vi "MGCC_LoadFcst_main.vi"() -> ()   [LabVIEW 2016]
uses:
  Sub-VIs/LoadCombinations.vi
  Sub-VIs/SW_Combinations.vi
  Sub-VIs/CriticalLoadIndex.vi
  <vilib>/imath/engines/lvmath2/RunTimeEngine/IndexRead/NIMS M($,S).vi
  <instcachedir>/0/NIMS M($,S)_3E5749BBB62E49528D4765A77F1F6D98.lvgen/NIMS M($,S)_3E5749BBB62E49528D4765A77F1F6D98_000.vi
  <vilib>/imath/engines/lvmath2/RunTimeEngine/BuiltInFunctions/findnz/NIMS_[1o]_findnz(GColV).vi
  <instcachedir>/0/NIMS_[1o]_findnz(GColV)_8556557C9365446B906472366DD9B2D8.lvgen/NIMS_[1o]_findnz(GColV)_8556557C9365446B906472366DD9B2D8_000.vi
  <vilib>/imath/engines/lvmath2/RunTimeEngine/BuiltInFunctions/length/NIMS_length(GV).vi
  <instcachedir>/0/NIMS_length(GV)_08A3D13377FD4E4B96F5795FBF3698FA.lvgen/NIMS_length(GV)_08A3D13377FD4E4B96F5795FBF3698FA_002.vi
  <vilib>/imath/engines/lvmath2/RunTimeEngine/ErrorHandling/NIMS_Create Error From Enums.vi
  <instcachedir>/0/NIMS_length(GV)_08A3D13377FD4E4B96F5795FBF3698FA.lvgen/NIMS_length(GV)_08A3D13377FD4E4B96F5795FBF3698FA_000.vi
  <vilib>/imath/engines/lvmath2/RunTimeEngine/BuiltInFunctions/zeros/NIMS_M=zeros(I32,I32).vi
  <vilib>/imathl/engines/lvmath/Functions/Error Handling/Create Error.vi
  <vilib>/imath/engines/lvmath2/RunTimeEngine/RangeToken/NIMS_Range_R2 - Integer.vi
  <instcachedir>/0/NIMS_Range_R2 - Integer_89B873E74E6E489885E44F751DD9C6BF.lvgen/NIMS_Range_R2 - Integer_89B873E74E6E489885E44F751DD9C6BF_000.vi
  <vilib>/imath/engines/lvmath2/RunTimeEngine/CommandStatement/MC_CommandStatement_break.vi
  <vilib>/imath/engines/lvmath2/RunTimeEngine/IndexRead/NIMS V(S).vi
  <instcachedir>/0/NIMS V(S)_0488751826AF41519A22953C041130DC.lvgen/NIMS V(S)_0488751826AF41519A22953C041130DC_000.vi
  <vilib>/imath/engines/lvmath2/RunTimeEngine/BuiltInFunctions/is_empty/NIMS_is_empty(GV).vi
  <instcachedir>/0/NIMS_is_empty(GV)_FC7E7C3D9544432CB6AA2416ADCF6D56.lvgen/NIMS_is_empty(GV)_FC7E7C3D9544432CB6AA2416ADCF6D56_000.vi
  <instcachedir>/0/NIMS V(S)_0488751826AF41519A22953C041130DC.lvgen/NIMS V(S)_0488751826AF41519A22953C041130DC_002.vi
  <vilib>/imath/engines/lvmath2/RunTimeEngine/IndexReplace/NIMS M(S,S)=S.vi
  <instcachedir>/0/NIMS M(S,S)=S_98E40400474E4398B113AE20298B4F82.lvgen/NIMS M(S,S)=S_98E40400474E4398B113AE20298B4F82_002.vi
  <vilib>/imath/engines/lvmath2/RunTimeEngine/NodeEndStatement/NIMS_NodeEndStatement_Output.vi
  <instcachedir>/0/NIMS_NodeEndStatement_Output_53EC0D466D134D7ABD903AC30B43404B.lvgen/NIMS_NodeEndStatement_Output_53EC0D466D134D7ABD903AC30B43404B_010.vi
  <vilib>/imath/engines/lvmath2/RunTimeEngine/ErrorHandling/NIMS_Finalize Error.vi
  Finite State Machine/Sub-VIs/MGCC_FntStaMach_gobal.vi
  <vilib>/Utility/error.llb/Error Cluster From Error Code.vi
  Communication/Global communication.vi
  Sub-VIs/Load_Mode.vi
  <vilib>/imath/engines/lvmath2/RunTimeEngine/Managers/WorkSpace/UID Generator.vi
  <vilib>/imath/engines/lvmath2/RunTimeEngine/ArithmeticOperatorToken/NIMS_ArithmeticOperator_times.vi
  <instcachedir>/0/NIMS_ArithmeticOperator_times_953B34F74CAC448FB707D816A29CC5F0.lvgen/NIMS_ArithmeticOperator_times_953B34F74CAC448FB707D816A29CC5F0_000.vi
  <vilib>/imath/engines/lvmath2/RunTimeEngine/ArithmeticOperatorToken/NIMS_ArithmeticOperator_multmx(M,CV).vi
  <instcachedir>/0/NIMS_ArithmeticOperator_multmx(M,CV)_EE734FC8520844C9A7CC1A67008668A3.lvgen/NIMS_ArithmeticOperator_multmx(M,CV)_EE734FC8520844C9A7CC1A67008668A3_001.vi
  <vilib>/imath/engines/lvmath2/RunTimeEngine/BuiltInFunctions/length/NIMS_length(GM).vi
  <instcachedir>/0/NIMS_length(GM)_47CEC356FCE0482D9BA47DC61C99F2C7.lvgen/NIMS_length(GM)_47CEC356FCE0482D9BA47DC61C99F2C7_000.vi
  <vilib>/imath/engines/lvmath2/RunTimeEngine/IndexRead/NIMS M(S).vi
  <instcachedir>/0/NIMS M(S)_B826C018497E4940AE96BD27B540B6FB.lvgen/NIMS M(S)_B826C018497E4940AE96BD27B540B6FB_000.vi
  <vilib>/imath/engines/lvmath2/RunTimeEngine/BuiltInFunctions/is_empty/NIMS_is_empty(GM).vi
  <instcachedir>/0/NIMS_is_empty(GM)_AF8F13F4B7FD436CB1855477E2504B8A.lvgen/NIMS_is_empty(GM)_AF8F13F4B7FD436CB1855477E2504B8A_004.vi
  <vilib>/imath/engines/lvmath2/RunTimeEngine/IndexReplace/NIMS M(S)=S.vi
  <instcachedir>/0/NIMS M(S)=S_B3274CDAFA9346529812A4A947D623CC.lvgen/NIMS M(S)=S_B3274CDAFA9346529812A4A947D623CC_001.vi
  <vilib>/imath/engines/lvmath2/RunTimeEngine/RunTimeType/NIMS_RunTimeType_From StrictType (excl LVString).vi
  <instcachedir>/0/NIMS_RunTimeType_From StrictType (excl LVString)_BBF44FB49F834B71AF7A14CCEDF8BECD.lvgen/NIMS_RunTimeType_From StrictType (excl LVString)_BBF44FB49F834B71AF7A14CCEDF8BECD_000.vi
  <vilib>/imath/engines/lvmath2/RunTimeEngine/LocalVariableDefStatement/MC_LocalVariableDefStatement_Display.vi
  <vilib>/imath/engines/lvmath2/RunTimeEngine/BuiltInFunctions/size/NIMS_[I32,I32]=size(GM).vi
  <instcachedir>/0/NIMS_[I32,I32]=size(GM)_B0A6EC1255BB4C8AB801FE6F734128D9.lvgen/NIMS_[I32,I32]=size(GM)_B0A6EC1255BB4C8AB801FE6F734128D9_000.vi
  <vilib>/imath/engines/lvmath2/RunTimeEngine/IndexRead/NIMS M(S,S).vi
  <instcachedir>/0/NIMS M(S,S)_AC51E74150A542F7991B9634C66F3096.lvgen/NIMS M(S,S)_AC51E74150A542F7991B9634C66F3096_000.vi
  <vilib>/imath/engines/lvmath2/RunTimeEngine/Managers/SymbolTable/Clear UID.vi
  <instcachedir>/0/NIMS_NodeEndStatement_Output_53EC0D466D134D7ABD903AC30B43404B.lvgen/NIMS_NodeEndStatement_Output_53EC0D466D134D7ABD903AC30B43404B_002.vi
  <vilib>/ErrorRing/Error Ring.xnode
  <vilib>/Analysis/NI_AALBase.lvlib
  <vilib>/imath/engines/lvmath2/RunTimeEngine/Managers/SymbolTable/NIMS_WorkSpace.lvlib
panel:
  out "SW_Combinations":i32[][](array[numeric])
  out "crit_index":i32[](array[numeric])
  out "Load_Combinations":i32[][](array[numeric])
  out "Default_L":dbl[](array[numeric])=[0.3, 0.5, 0.2, 0.27, 0.25, 0.2, 0.18]
  out "Forecast":dbl[][](graph)
  out "Weekend_History":dbl[][](graph)
  out "Weekday_History":dbl[][](graph)
  out "err1":errorcluster
  out "f_MGCC_LoadFcst_FcstLoad":dbl[][](array[numeric])
  # "Copyright <2020> <The University of Tennessee at Knoxville and the University of Tennessee Research Foundation>\n\nRedistribution and use in source and binary forms, with or without modification, are permitted provided that the following conditions are met:\n\n1. Redistributions of source code must retain the above copyright notice, this list of conditions and the following disclaimer.\n\n2. Redistributions in binary form must reproduce the above copyright notice, this list of conditions and the following disclaimer in the documentation and/or other materials provided with the distribution.\n\n3. Neither the name of the copyright holder nor the names of its contributors may be used to endorse or promote products derived from this software without specific prior written permission.\n\nTHIS SOFTWARE IS PROVIDED BY THE COPYRIGHT HOLDERS AND CONTRIBUTORS \"AS IS\" AND ANY EXPRESS OR IMPLIED WARRANTIES, INCLUDING, BUT NOT LIMITED TO, THE IMPLIED WARRANTIES OF MERCHANTABILITY AND FITNESS FOR A PARTICULAR PURPOSE ARE DISCLAIMED. IN NO EVENT SHALL THE COPYRIGHT HOLDER OR CONTRIBUTORS BE LIABLE FOR ANY DIRECT, INDIRECT, INCIDENTAL, SPECIAL, EXEMPLARY, OR CONSEQUENTIAL DAMAGES (INCLUDING, BUT NOT LIMITED TO, PROCUREMENT OF SUBSTITUTE GOODS OR SERVICES; LOSS OF USE, DATA, OR PROFITS; OR BUSINESS INTERRUPTION) HOWEVER CAUSED AND ON ANY THEORY OF LIABILITY, WHETHER IN CONTRACT, STRICT LIABILITY, OR TORT (INCLUDING NEGLIGENCE OR OTHERWISE) ARISING IN ANY WAY OUT OF THE USE OF THIS SOFTWARE, EVEN IF ADVISED OF THE POSSIBILITY OF SUCH DAMAGE."
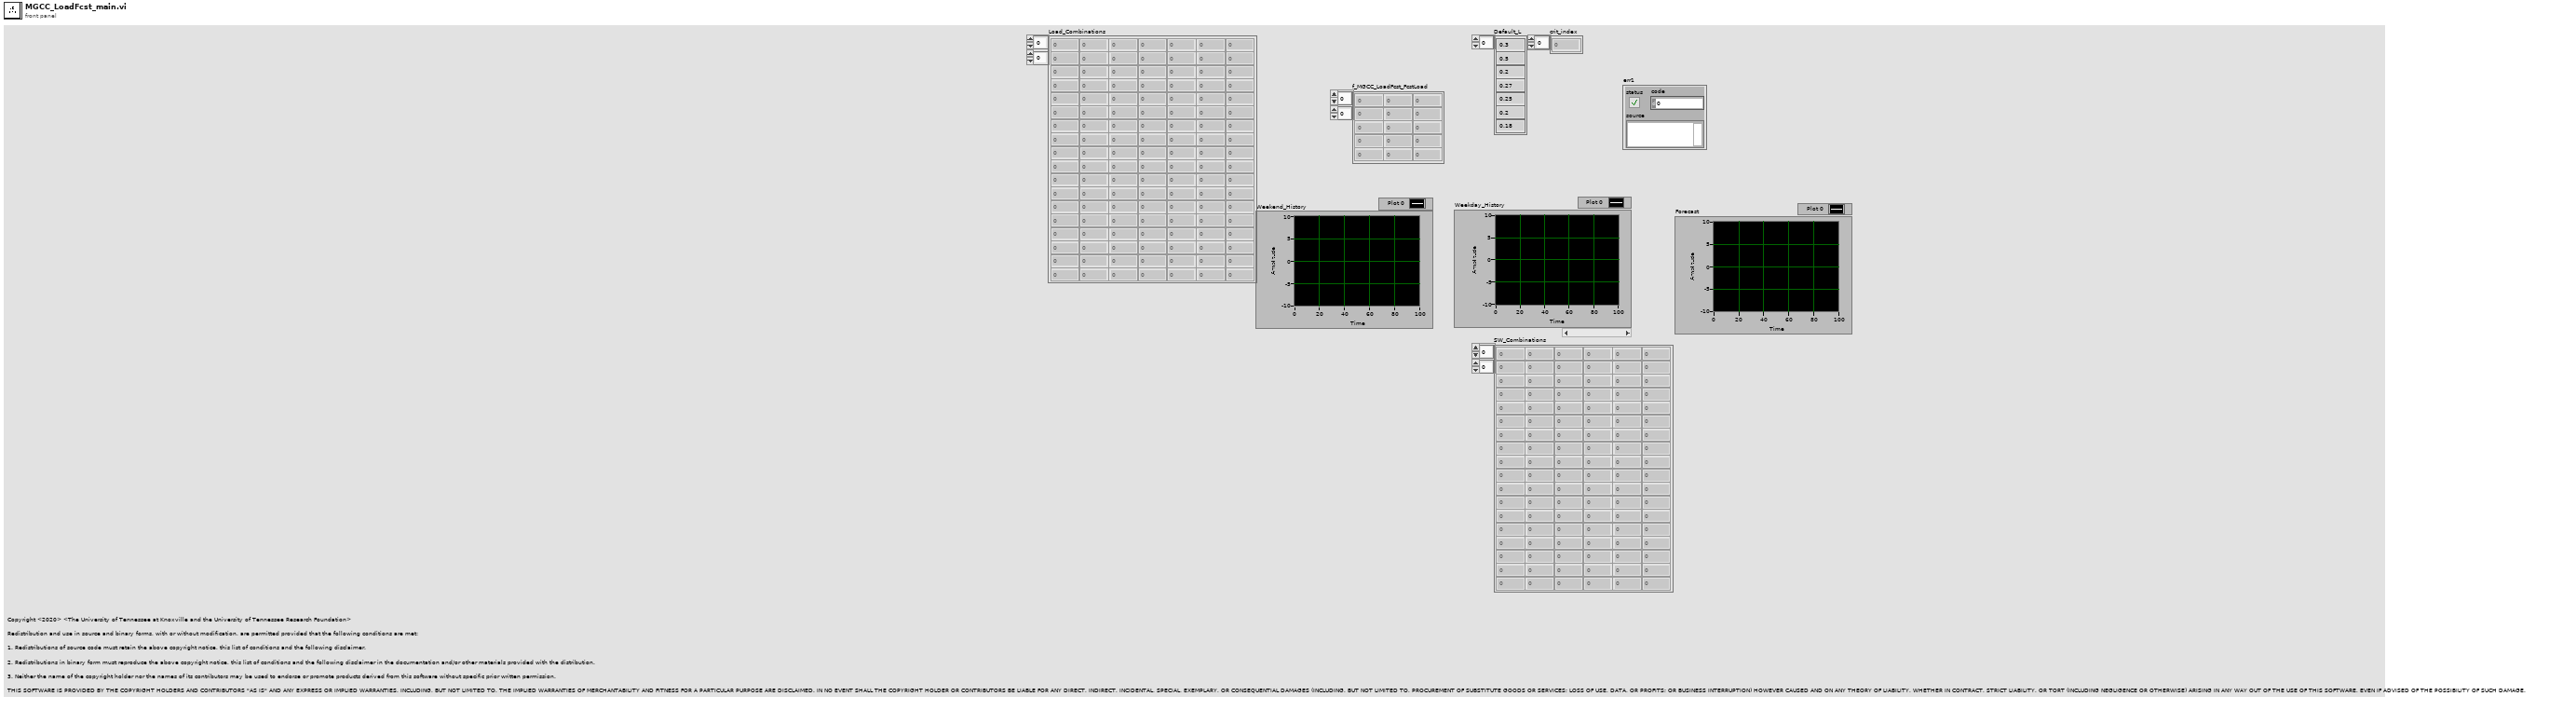
[diagram p1: front panel]
types:
  T1 = typedef "NI_Matrix.lvlib/RealMatrix.ctl" = dbl[][]
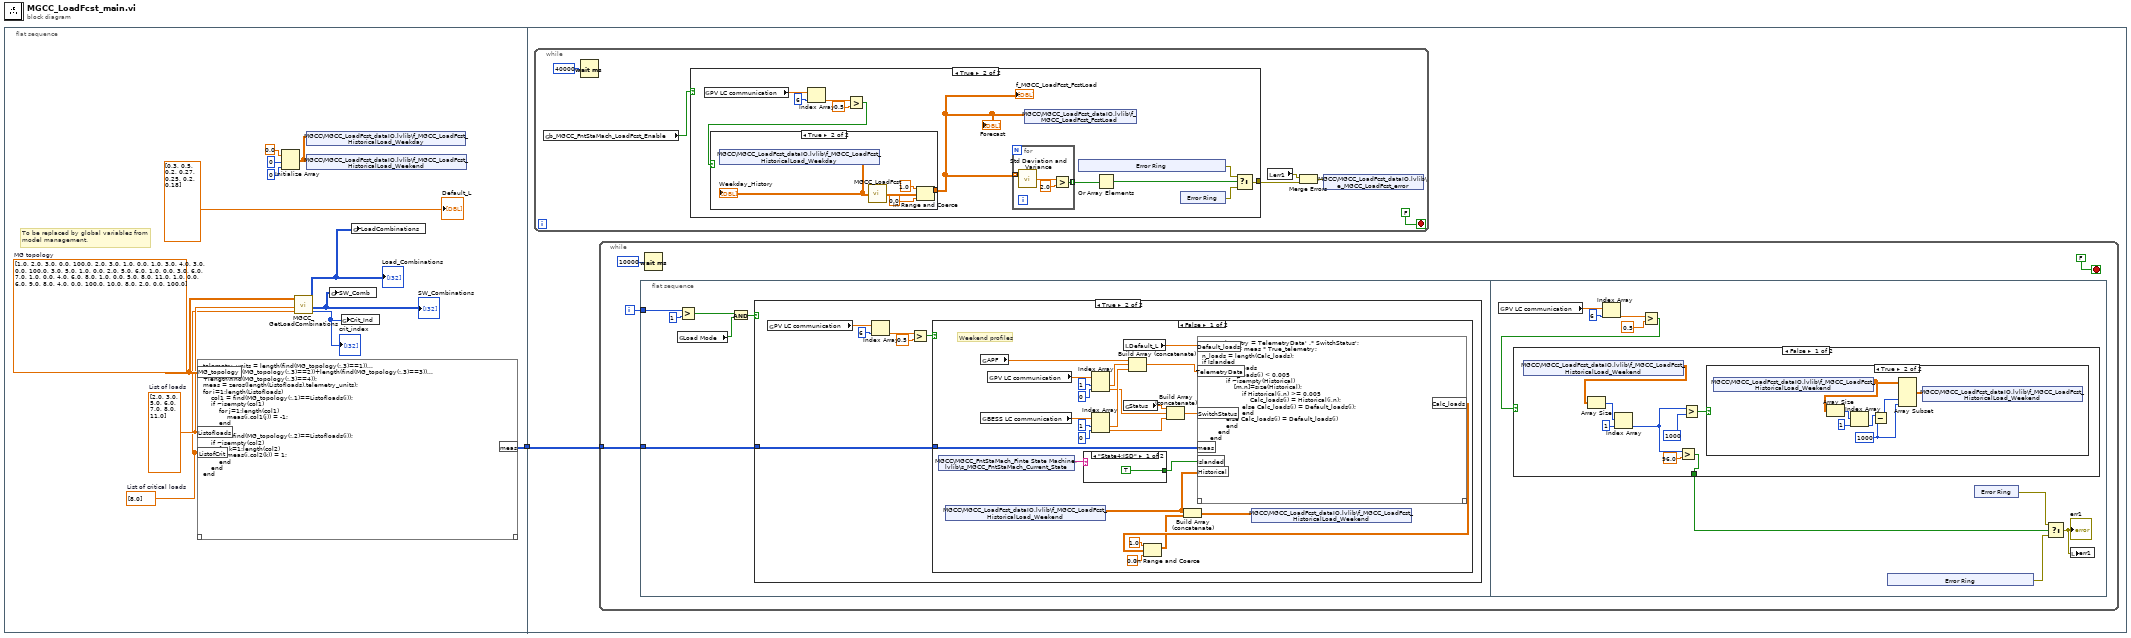
[diagram p0: block diagram]
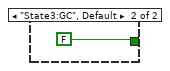
[diagram p3: hidden frame]
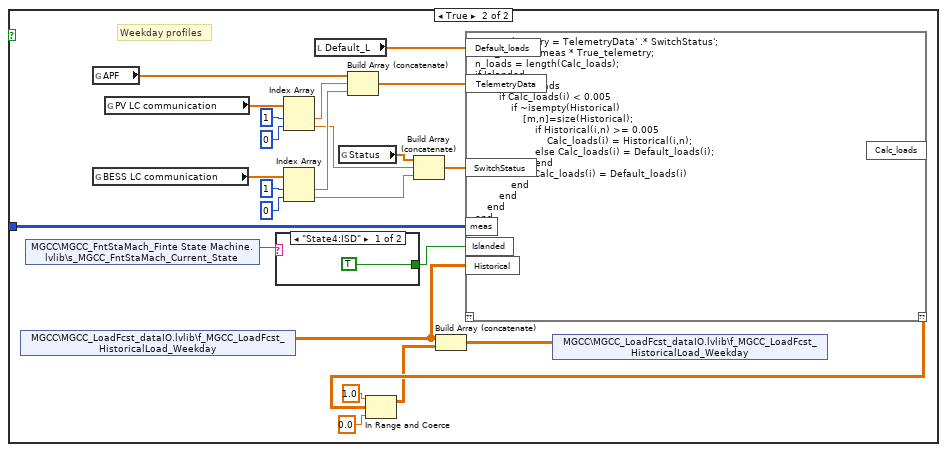
[diagram p4: hidden frame]
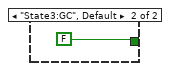
[diagram p5: hidden frame]
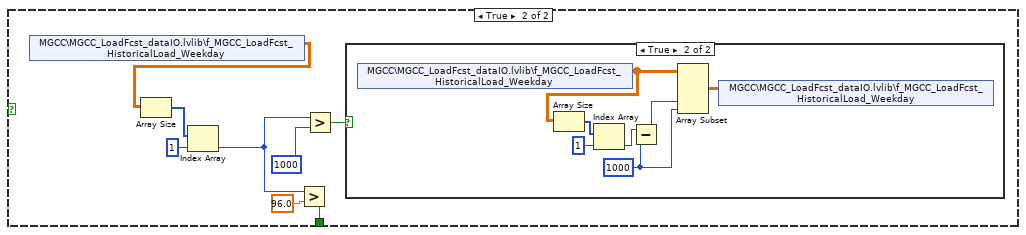
[diagram p7: hidden frame]
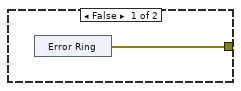
[diagram p9: hidden frame]
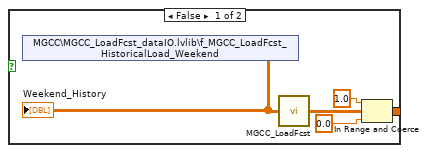
[diagram p10: hidden frame]
diagram:
  n1 = flat-sequence {
    tunnel: [w9] -> w1
    tunnel: w1 -> [w389]
    frame #0 {
      w5 = dbl[] [8.0]  # List of critical loads
      w6 = dbl[] [2.0, 3.0, 5.0, 6.0, 7.0, 8.0, 11.0]  # List of loads
      w7 = dbl[][] [[1.0, 2.0, 3.0, 0.0, 100.0], [2.0, 3.0, 1.0, 0.0, 1.0], [3.0, 4.0, 3.0, 0.0, 100.0], [3.0, 5.0, 1.0, 0.0, 2.0], [5.0, 6.0, 1.0, 0.0, 3.0], [6.0, 7.0, 1.0, 0.0, 4.0], [6.0, 8.0, 1.0, 0.0, 5.0], [8.0, 11.0, 1.0, 0.0, 6.0], [9.0, 8.0, 4.0, 0.0, 100.0], [10.0, 8.0, 2.0, 0.0, 100.0]]  # MG topology
      # "To be replaced by global variables from model management."
      n2 = mathscript code="telemetry_units = length(find(MG_topology(:,3)==1))...\n+length(find(MG_topology(:,3)==2))+length(find(MG_topology(:,3)==3))...\n+length(find(MG_topology(:,3)==4));\nmeas = zeros(length(Listofloads),telemetry_units);\nfor i=1:length(Listofloads)\n    col1 = find(MG_topology(:,1)==Listofloads(i));\n    if ~isempty(col1)\n        for j=1:length(col1)\n            meas(i,col1(j)) = -1;\n        end\n    end\n    col2 = find(MG_topology(:,2)==Listofloads(i));\n    if ~isempty(col2)\n        for k=1:length(col2)\n            meas(i,col2(k)) = 1;\n        end\n    end\nend"("MG_topology"=w7, "Listofloads"=w6, "ListofCrit"=w5) -> ("meas"=w9:i32[][])  [unwired: 1 in, 1 out]
      n3 = Initialize Array(0.0 ("element"), 0 ("dimension size"), 0 ("dimension size")) -> (w10:dbl[][])
      n4 = call "MGCC_GetLoadCombinations.vi"("List pf critical loads"=w5, "List of loads"=w6, "MG topology"=w7) -> ("crit_index"=w3:i32[], "ValidComb"=w2:i32[][], "Load_Combinations"=w4:i32[][])  [unwired: 6 in]
      "Load_Combinations" <- w4
      "crit_index" <- w3
      "SW_Combinations" <- w2
      n5 = shared-variable "MGCC\\MGCC_LoadFcst_dataIO.lvlib\\f_MGCC_LoadFcst_HistoricalLoad_Weekday"(w10) -> ()  [unwired: 1 in, 1 out]
      n6 = shared-variable "MGCC\\MGCC_LoadFcst_dataIO.lvlib\\f_MGCC_LoadFcst_HistoricalLoad_Weekend"(w10) -> ()  [unwired: 1 in, 1 out]
      n7 = global write "SW_Combinations.vi" "SW_Comb"(w2) -> ()
      n8 = global write "CriticalLoadIndex.vi" "Crit_Ind"(w3) -> ()
      n9 = global write "LoadCombinations.vi" "LoadCombinations"(w4) -> ()
      "Default_L" <- dbl[] [0.3, 0.5, 0.2, 0.27, 0.25, 0.2, 0.18]
    }
    frame #1 {
      n10 = while {
        stop <- FALSE stop-if-true
        n11 = global read "MGCC_FntStaMach_gobal.vi" "b_MGCC_FntStaMach_LoadFcst_Enable"() -> (w1185:bool)
        n12 = Wait (ms)(milliseconds to wait=u32 40000) -> ()  [unwired: 1 out]
        n13 = case shown="True" w1185 {
          tunnel: [w1191 w1201] -> w1188
          frame False {
            n14 = xnode "Error Ring"() -> ("error out"=w1191:errorcluster)
          }
          frame True {
            n15 = global read "Global communication.vi" "PV LC communication"() -> (w1200:dbl[])
            n16 = Index Array(array=w1200, index=6) -> (element=w1198:dbl)
            n17 = Greater?(x=w1198, y=0.5) -> (0:w1196:bool)
            n18 = case shown="True" w1196 {
              tunnel: [w1208 w1213] -> w1195
              frame False {
                n19 = shared-variable "MGCC\\MGCC_LoadFcst_dataIO.lvlib\\f_MGCC_LoadFcst_HistoricalLoad_Weekend"() -> (w1211:dbl[][])  [unwired: 1 in, 1 out]
                "Weekend_History" <- w1211
                n20 = call "MGCC_LoadFcst.vi"("InputTimeSeries"=w1211) -> ("OutputTimeSeries"=w1212:dbl[][])
                n21 = In Range and Coerce(upper limit=1.0, x=w1212, lower limit=0.0) -> (coerced(x)=w1208:dbl[][])  [unwired: 1 out]
              }
              frame True {
                n22 = shared-variable "MGCC\\MGCC_LoadFcst_dataIO.lvlib\\f_MGCC_LoadFcst_HistoricalLoad_Weekday"() -> (w1216:dbl[][])  [unwired: 1 in, 1 out]
                "Weekday_History" <- w1216
                n23 = call "MGCC_LoadFcst.vi"("InputTimeSeries"=w1216) -> ("OutputTimeSeries"=w1217:dbl[][])
                n24 = In Range and Coerce(upper limit=1.0, x=w1217, lower limit=0.0) -> (coerced(x)=w1213:dbl[][])  [unwired: 1 out]
              }
            }
            "f_MGCC_LoadFcst_FcstLoad" <- w1195
            "Forecast" <- w1195
            n25 = for {
              tunnel: w1195 -> [w1205] mode=indexing
              tunnel: [w1204] -> w1194 mode=indexing
              n26 = call <vilib>:"Std Deviation and Variance.vi"("X"=w1205) -> ("standard deviation"=w1207:dbl)  [unwired: 1 in, 2 out]
              n27 = Greater?(x=w1207, y=2.0) -> (0:w1204:bool)
            }
            n28 = shared-variable "MGCC\\MGCC_LoadFcst_dataIO.lvlib\\f_MGCC_LoadFcst_FcstLoad"(w1195) -> ()  [unwired: 1 in, 1 out]
            n29 = xnode "Error Ring"() -> ("error out"=w1202:errorcluster)
            n30 = Or Array Elements(Boolean array=w1194) -> (logical OR=w1193:bool)
            n31 = xnode "Error Ring"() -> ("error out"=w1203:errorcluster)
            n32 = Select(t=w1202, s=w1193, f=w1203) -> (s? t:f=w1201:errorcluster)
          }
        }
        n33 = local read "err1"() -> (w1186:errorcluster)
        n34 = Merge Errors(w1186, w1188) -> (w1187:errorcluster)
        n35 = shared-variable "MGCC\\MGCC_LoadFcst_dataIO.lvlib\\e_MGCC_LoadFcst_error"(w1187) -> ()  [unwired: 1 in, 1 out]
      }
      n36 = while {
        tunnel: w389 -> [w390]
        i -> [w391]
        stop <- FALSE stop-if-true
        n37 = flat-sequence {
          tunnel: w391 -> [w399]
          tunnel: w390 -> [w394]
          frame #0 {
            n38 = global read "Load_Mode.vi" "Load Mode"() -> (w397:bool)
            n39 = Greater?(x=w399, y=1) -> (0:w396:bool)
            n40 = And(x=w396, y=w397) -> (x .and. y?=w395:bool)
            n41 = case shown="True" w395 {
              tunnel: w394 -> [_ w400]
              frame False {
              }
              frame True {
                n42 = global read "Global communication.vi" "PV LC communication"() -> (w405:dbl[])
                n43 = Index Array(array=w405, index=6) -> (element=w403:dbl)
                n44 = Greater?(x=w403, y=0.5) -> (0:w401:bool)
                n45 = case shown="False" w401 {
                  tunnel: w400 -> [w410 w782]
                  frame False {
                    # "Weekend profiles"
                    n46 = shared-variable "MGCC\\MGCC_FntStaMach_Finte State Machine.lvlib\\s_MGCC_FntStaMach_Current_State"() -> (w409:string)  [unwired: 1 in, 1 out]
                    n47 = shared-variable "MGCC\\MGCC_LoadFcst_dataIO.lvlib\\f_MGCC_LoadFcst_HistoricalLoad_Weekend"() -> (w407:dbl[][])  [unwired: 1 in, 1 out]
                    n48 = global read "Global communication.vi" "APF"() -> (w423:dbl[])
                    n49 = global read "Global communication.vi" "BESS LC communication"() -> (w428:dbl[])
                    n50 = global read "Global communication.vi" "PV LC communication"() -> (w429:dbl[])
                    n51 = case shown="\"State4:ISD\"" w409 {
                      tunnel: [TRUE FALSE] -> w408
                      frame "State4:ISD" {
                      }
                      frame "State3:GC", Default {
                      }
                    }
                    n52 = Index Array(array=w429, index #1=1 ("index"), index #2=0 ("index")) -> (element #1=w422:dbl, element #2=w419:dbl)
                    n53 = Index Array(array=w428, index #1=1 ("index"), index #2=0 ("index")) -> (element #1=w421:dbl, element #2=w418:dbl)
                    n54 = local read "Default_L"() -> (w406:dbl[])
                    n55 = global read "Global communication.vi" "Status"() -> (w420:dbl[])
                    n56 = Build Array (concatenate)(w423, w422, w421) -> (w417:dbl[])
                    n57 = Build Array (concatenate)(w420, w419, w418) -> (w416:dbl[])
                    n58 = mathscript code="True_telemetry = TelemetryData' .* SwitchStatus';\nCalc_loads = meas * True_telemetry;\nn_loads = length(Calc_loads);\nif Islanded\n    for i=1:n_loads\n        if Calc_loads(i) < 0.005\n            if ~isempty(Historical)\n                [m,n]=size(Historical);\n                    if Historical(i,n) >= 0.005\n                        Calc_loads(i) = Historical(i,n);\n                    else Calc_loads(i) = Default_loads(i);\n                    end\n            else Calc_loads(i) = Default_loads(i)\n            end\n        end\n    end\nend"("TelemetryData"=w417, "SwitchStatus"=w416, "meas"=w410, "Islanded"=w408, "Historical"=w407, "Default_loads"=w406) -> ("Calc_loads"=w415:dbl[][])  [unwired: 1 in, 1 out]
                    n59 = In Range and Coerce(upper limit=1.0, x=w415, lower limit=0.0) -> (coerced(x)=w412:dbl[][])  [unwired: 1 out]
                    n60 = Build Array (concatenate)(w407, w412) -> (w411:T1)
                    n61 = shared-variable "MGCC\\MGCC_LoadFcst_dataIO.lvlib\\f_MGCC_LoadFcst_HistoricalLoad_Weekend"(w411) -> ()  [unwired: 1 in, 1 out]
                  }
                  frame True {
                    # "Weekday profiles"
                    n62 = shared-variable "MGCC\\MGCC_LoadFcst_dataIO.lvlib\\f_MGCC_LoadFcst_HistoricalLoad_Weekday"() -> (w774:dbl[][])  [unwired: 1 in, 1 out]
                    n63 = shared-variable "MGCC\\MGCC_FntStaMach_Finte State Machine.lvlib\\s_MGCC_FntStaMach_Current_State"() -> (w776:string)  [unwired: 1 in, 1 out]
                    n64 = global read "Global communication.vi" "APF"() -> (w790:dbl[])
                    n65 = global read "Global communication.vi" "BESS LC communication"() -> (w795:dbl[])
                    n66 = global read "Global communication.vi" "PV LC communication"() -> (w796:dbl[])
                    n67 = case shown="\"State4:ISD\"" w776 {
                      tunnel: [TRUE FALSE] -> w775
                      frame "State4:ISD" {
                      }
                      frame "State3:GC", Default {
                      }
                    }
                    n68 = Index Array(array=w796, index #1=1 ("index"), index #2=0 ("index")) -> (element #1=w789:dbl, element #2=w786:dbl)
                    n69 = Index Array(array=w795, index #1=1 ("index"), index #2=0 ("index")) -> (element #1=w788:dbl, element #2=w785:dbl)
                    n70 = local read "Default_L"() -> (w773:dbl[])
                    n71 = global read "Global communication.vi" "Status"() -> (w787:dbl[])
                    n72 = Build Array (concatenate)(w790, w789, w788) -> (w784:dbl[])
                    n73 = Build Array (concatenate)(w787, w786, w785) -> (w783:dbl[])
                    n74 = mathscript code="True_telemetry = TelemetryData' .* SwitchStatus';\nCalc_loads = meas * True_telemetry;\nn_loads = length(Calc_loads);\nif Islanded\n    for i=1:n_loads\n        if Calc_loads(i) < 0.005\n            if ~isempty(Historical)\n                [m,n]=size(Historical);\n                    if Historical(i,n) >= 0.005\n                        Calc_loads(i) = Historical(i,n);\n                    else Calc_loads(i) = Default_loads(i);\n                    end\n            else Calc_loads(i) = Default_loads(i)\n            end\n        end\n    end\nend"("TelemetryData"=w784, "SwitchStatus"=w783, "meas"=w782, "Islanded"=w775, "Historical"=w774, "Default_loads"=w773) -> ("Calc_loads"=w781:dbl[][])  [unwired: 1 in, 1 out]
                    n75 = In Range and Coerce(upper limit=1.0, x=w781, lower limit=0.0) -> (coerced(x)=w778:dbl[][])  [unwired: 1 out]
                    n76 = Build Array (concatenate)(w774, w778) -> (w777:T1)
                    n77 = shared-variable "MGCC\\MGCC_LoadFcst_dataIO.lvlib\\f_MGCC_LoadFcst_HistoricalLoad_Weekday"(w777) -> ()  [unwired: 1 in, 1 out]
                  }
                }
              }
            }
          }
          frame #1 {
            n78 = global read "Global communication.vi" "PV LC communication"() -> (w1144:dbl[])
            n79 = Index Array(array=w1144, index=6) -> (element=w1142:dbl)
            n80 = Greater?(x=w1142, y=0.5) -> (0:w1140:bool)
            n81 = case shown="False" w1140 {
              tunnel: [w1149 w1168] -> w1148
              frame False {
                n82 = shared-variable "MGCC\\MGCC_LoadFcst_dataIO.lvlib\\f_MGCC_LoadFcst_HistoricalLoad_Weekend"() -> (w1153:dbl[][])  [unwired: 1 in, 1 out]
                n83 = Array Size(array=w1153) -> (size(s)=w1152:i32[])
                n84 = Index Array(array=w1152, index=1) -> (element=w1150:i32)
                n85 = Greater?(x=w1150, y=96.0) -> (0:w1149:bool)
                n86 = Greater?(x=w1150, y=1000) -> (0:w1156:bool)
                n87 = case shown="True" w1156 {
                  frame False {
                  }
                  frame True {
                    w1158 = 1000 ("y")
                    n88 = shared-variable "MGCC\\MGCC_LoadFcst_dataIO.lvlib\\f_MGCC_LoadFcst_HistoricalLoad_Weekend"() -> (w1163:dbl[][])  [unwired: 1 in, 1 out]
                    n89 = Array Size(array=w1163) -> (size(s)=w1162:i32[])
                    n90 = Index Array(array=w1162, index=1) -> (element=w1160:i32)
                    n91 = Subtract(x=w1160, y=w1158) -> (x-y=w1159:i32)
                    n92 = Array Subset(array=w1163, index (col)=w1159, length (col)=w1158) -> (w1157:dbl[][])  [unwired: 2 in]
                    n93 = shared-variable "MGCC\\MGCC_LoadFcst_dataIO.lvlib\\f_MGCC_LoadFcst_HistoricalLoad_Weekend"(w1157) -> ()  [unwired: 1 in, 1 out]
                  }
                }
              }
              frame True {
                n94 = shared-variable "MGCC\\MGCC_LoadFcst_dataIO.lvlib\\f_MGCC_LoadFcst_HistoricalLoad_Weekday"() -> (w1167:dbl[][])  [unwired: 1 in, 1 out]
                n95 = Array Size(array=w1167) -> (size(s)=w1166:i32[])
                n96 = Index Array(array=w1166, index=1) -> (element=w1164:i32)
                n97 = Greater?(x=w1164, y=96.0) -> (0:w1168:bool)
                n98 = Greater?(x=w1164, y=1000) -> (0:w1171:bool)
                n99 = case shown="True" w1171 {
                  frame False {
                  }
                  frame True {
                    w1173 = 1000 ("y")
                    n100 = shared-variable "MGCC\\MGCC_LoadFcst_dataIO.lvlib\\f_MGCC_LoadFcst_HistoricalLoad_Weekday"() -> (w1178:dbl[][])  [unwired: 1 in, 1 out]
                    n101 = Array Size(array=w1178) -> (size(s)=w1177:i32[])
                    n102 = Index Array(array=w1177, index=1) -> (element=w1175:i32)
                    n103 = Subtract(x=w1175, y=w1173) -> (x-y=w1174:i32)
                    n104 = Array Subset(array=w1178, index (col)=w1174, length (col)=w1173) -> (w1172:dbl[][])  [unwired: 2 in]
                    n105 = shared-variable "MGCC\\MGCC_LoadFcst_dataIO.lvlib\\f_MGCC_LoadFcst_HistoricalLoad_Weekday"(w1172) -> ()  [unwired: 1 in, 1 out]
                  }
                }
              }
            }
            n106 = xnode "Error Ring"() -> ("error out"=w1146:errorcluster)
            n107 = xnode "Error Ring"() -> ("error out"=w1147:errorcluster)
            n108 = Select(t=w1147, s=w1148, f=w1146) -> (s? t:f=w1145:errorcluster)
            "err1" <- w1145
            n109 = local write "err1"(w1145) -> ()
          }
        }
        n110 = Wait (ms)(milliseconds to wait=u32 10000) -> ()  [unwired: 1 out]
      }
    }
  }
